vi "Process.vi"(8 "error in":errorcluster, 11 "SMO":refnum<class "SMO.lvclass">) -> (0 "error out":errorcluster, 3 "SMO out":refnum<class "SMO.lvclass">)   [LabVIEW 2013, in "SMO.lvclass"]
uses:
  SMO.lvclass
panel:
  # "For instructions on how to use the JKI State Machine Objects, examples and video tutorials, visit:\nhttp://jki.net/state-machine-objects/\n\nJKI State Machine Objects™\nhttp://jki.net/state-machine-objects/\nCopyright (C) 2005-2015, JKI <info@jki.net>\nALL RIGHTS RESERVED"
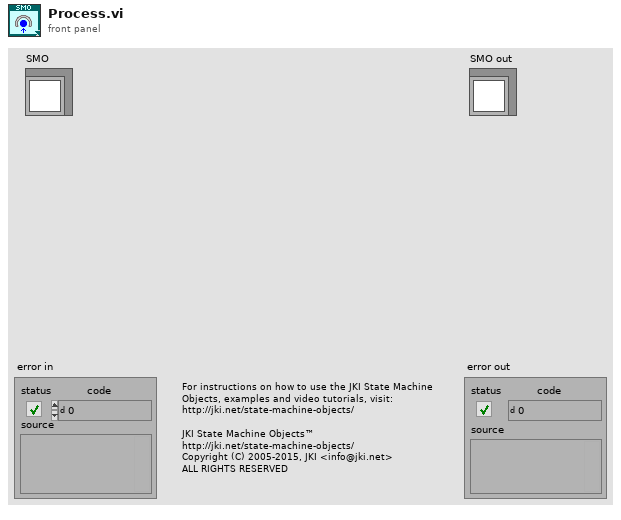
[diagram p1: front panel]
types:
  T1 = typedef "SMO.lvclass/Parent Call--Enum.ctl" = enum16{"Allows parent to run", "Does not request parent to run"}
  T2 = typedef "SMO.lvclass/Protected Events.ctl" = cluster{"StopProcesses":refnum<user-event>, "AbortProcesses":refnum<user-event>}
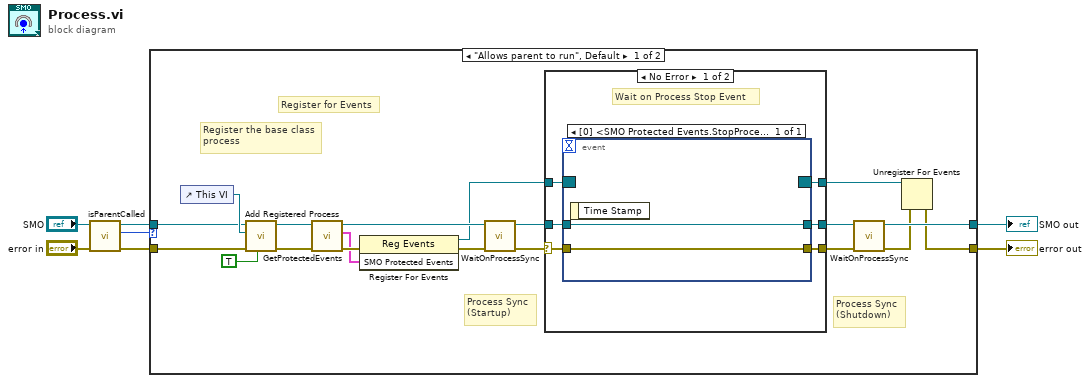
[diagram p0: block diagram]
diagram:
  n1 = call "isParentCalled.vi"("error in (no error)"="error in", "SMO in"="SMO") -> ("error out"=w2:errorcluster, "Parent Call"=w1:T1, "SMO out"=w4:refnum<class "SMO.lvclass">)  [unwired: 7 in]
  n2 = case shown="\"Allows parent to run\", Default" w1 {
    tunnel: [w22 w39] -> w7
    tunnel: [w19 w38] -> w6
    tunnel: w4 -> [w11 w39]
    tunnel: w2 -> [w10 w38]
    frame "Allows parent to run", Default {
      # "Register the base class\nprocess"
      # "Process Sync\n(Shutdown)"
      # "Process Sync\n(Startup)"
      # "Register for Events"
      n3 = control-ref of="This VI"() -> (w13:refnum<vi>)
      n4 = call "Add Registered Process.vi"("Process Runs (T)"=TRUE, "error in (no error)"=w10, "Process VI (Static VI Ref)"=w13, "SMO"=w11) -> ("error out"=w14:errorcluster, "SMO out"=w15:refnum<class "SMO.lvclass">)  [unwired: 6 in]
      n5 = call "GetProtectedEvents.vi"("error in (no error)"=w14, "SMO"=w15) -> ("error out"=w17:errorcluster, "SMO Protected Events"=w12:T2, "SMO out"=w26:refnum<class "SMO.lvclass">)  [unwired: 7 in]
      n6 = register-events(error in=w17, w12) -> (reference out=w18:refnum<event-registration>, error out=w16:errorcluster)  [unwired: 1 in]
      n7 = call "WaitOnProcessSync.vi"("error in (no error)"=w16, "SMO"=w26) -> ("error out"=w8:errorcluster, "SMO out"=w25:refnum<class "SMO.lvclass">)  [unwired: 8 in]
      n8 = case shown="No Error" w8 {
        selector: w8 -> [w27 w35]
        tunnel: w25 -> [w32 w36]
        tunnel: [w31 w35] -> w24
        tunnel: [w30 w36] -> w23
        tunnel: [w29 w37] -> w21
        tunnel: w18 -> [w28 w37]
        frame No Error {
          # "Wait on Process Stop Event"
          n9 = event shown="[0] <SMO Protected Events.StopProcesses>, <SMO Protected Events.AbortProcesses>: User Event" {
            selector: w28 -> [_]
            dyn-events: [_] -> w29
            timeout: _ -> [_]
            tunnel: w32 -> [w33]
            tunnel: w27 -> [w34]
            tunnel: [w34] -> w31
            tunnel: [w33] -> w30
            event User Event {
              n10 = event-data() -> ()  [unwired: 1 in, 1 out]
            }
          }
        }
        frame Error {
        }
      }
      n11 = call "WaitOnProcessSync.vi"("error in (no error)"=w24, "SMO"=w23) -> ("error out"=w20:errorcluster, "SMO out"=w22:refnum<class "SMO.lvclass">)  [unwired: 8 in]
      n12 = Unregister For Events(event registration refnum=w21, error in=w20) -> (error out=w19:errorcluster)
    }
    frame "Does not request parent to run" {
    }
  }
  "error out" <- w6
  "SMO out" <- w7
